vi "Write formula_info.vi"(8 "error in (no error)":errorcluster, 10 "formula_info":cluster{"Table":i32[][], "Y Values":dbl[]} {"Y Values" format="%.2f"}, 11 "Alicat_P in":refnum<class "P.lvclass">) -> (0 "error out":errorcluster, 3 "Alicat_P out":refnum<class "P.lvclass">)   [LabVIEW 2015, in "Alicat.lvlib" / "P.lvclass"]
uses:
  P.lvclass
  P.lvclass/P.ctl
panel:
  # "operator"
  # "register1"
  # "register2"
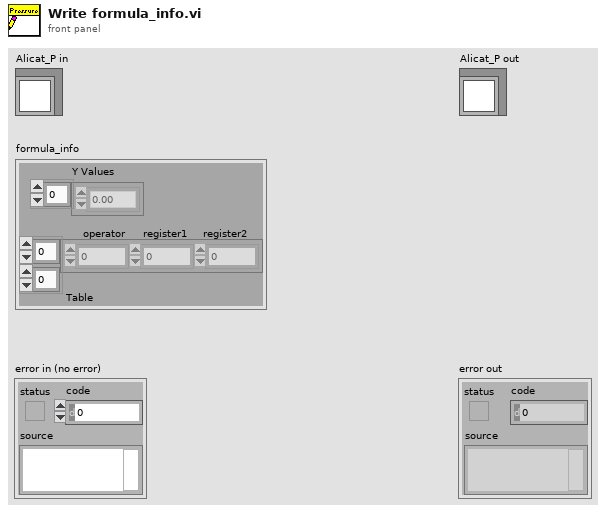
[diagram p1: front panel]
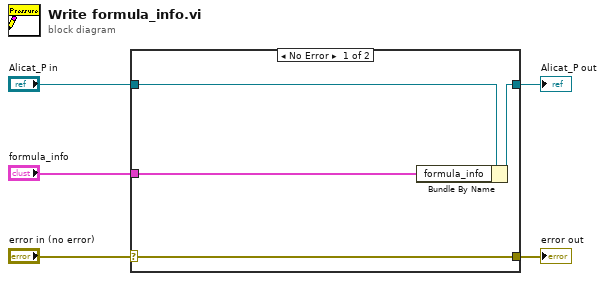
[diagram p0: block diagram]
diagram:
  n1 = case shown="No Error" "error in (no error)" {
    selector: "error in (no error)" -> [w9 w10]
    tunnel: [w9 w10] -> w4
    tunnel: [w7 w11] -> w2
    tunnel: "Alicat_P in" -> [w8 w11]
    tunnel: "formula_info" -> [w6 _]
    frame No Error {
      n2 = Bundle By Name(cluster=w8, "formula_info"=w6) -> (w7:refnum<class "P.lvclass">)
    }
    frame Error {
    }
  }
  "error out" <- w4
  "Alicat_P out" <- w2
